vi "IV_Reader.vi"(7 "Path to PNG Folder":path, 8 "Use only a subset of the folder":bool=TRUE, 9 "Subset Length":i32, 10 "Subset Index":i32, 11 "Folder or File":path=path "B:/SketchSET/SA03008H.20180718/08-BG_Sweep_-5to5_0.1_@0.1Hz") -> ()   [LabVIEW 2016]
uses:
  <userlib>/LevyLab/LV to ITX/LVtoITX.lvclass
  <vilib>/Analysis/NI_AALBase.lvlib
  <vilib>/Analysis/1siggen.llb/Ramp Pattern by Delta.vi
  <vilib>/MakerHub/Toolbox/LMH-Toolbox.lvlib
panel:
  in  "dI/dV OFFSET":dbl=100.0 format="%#_13g"
  in  "IV OFFSET":dbl=2e-10 format="%#_13g"
  in  "e^2/h ?":bool
  in  "X step":dbl
  in  "X start":dbl
  out "Differential Conductance":dbl[][](graph)=[[172.002], [172.014], [172.02], [172.032], [172.05], [172.038], [171.99], [171.984], [172.008], [172.02], [172.038], [172.032], [172.008], [171.99], [171.984], [171.99], [172.008], [172.02], [172.032], [171.996], [172.002], [172.014], [172.032], [172.056], [172.056], [172.038], [172.008], [171.996], [172.014], [172.026], [172.032], [172.044], [172.008], [171.996], [171.99], [172.014], [172.032], [172.038], [172.032], [171.99], [171.984], [171.996], [172.014], [172.032], [172.026], [172.002], [171.99], [171.996], [172.02], [172.038], [172.05], [172.032], [172.002], [172.008], [172.014], [172.032], [172.044], [172.056], [172.044], [172.002], [171.996], [172.002], [172.026], [172.038], [172.044], [172.05], [172.02], [172.002], [171.99], [172.002], [172.008], [172.026], [172.02], [171.978], [171.978], [171.984], [171.99], [171.99], [172.002], [171.978], [171.96], [171.972], [171.984], [171.99], [171.996], [171.996], [171.978], [171.954], [171.948], [171.972], [171.99], [172.008], [172.032], [172.014], [171.996], [172.008], [172.014], [172.014], [172.008], [171.99], [171.972], [171.972], [171.99], [172.008], [172.032], [172.02], [171.996], [171.984], [171.996], [172.014], [172.02], [172.002], [171.972], [171.978], [171.99], [172.008], [172.026], [172.026], [171.99], [171.978], [171.99], [171.996], [172.002], [172.002], [172.002]]
  in  "Portion of data":cluster{dbl, dbl}(slide)={0.75, 0.25} scale=0.0..1.0
  out "hmmmm":cluster{dbl[], dbl[]}(graph)
  out "Iterations of loop":i32
  out "directory":bool
  out "dI/dV":cluster{dbl[], dbl[]}[](graph)
  out "A vs B":cluster{dbl[], dbl[]}[](graph)
  in  "Diff bin size":dbl
  out "Comments":string
  in  "Diff bin size":dbl=2.0
  out "N__":cluster{"N1":dbl, "N2":dbl, "N3":dbl, "N4":dbl}={"N1"=0.0624995231628418, "N2"=0.0624995231628418, "N3"=0.0624995231628418, "N4"=0.0624995231628418} {"N4" format="%#_6p"; "N3" format="%#_6p"; "N2" format="%#_6p"; "N1" format="%#_6p"}
  out "IV":dbl[][](graph)=[[172.002], [172.014], [172.02], [172.032], [172.05], [172.038], [171.99], [171.984], [172.008], [172.02], [172.038], [172.032], [172.008], [171.99], [171.984], [171.99], [172.008], [172.02], [172.032], [171.996], [172.002], [172.014], [172.032], [172.056], [172.056], [172.038], [172.008], [171.996], [172.014], [172.026], [172.032], [172.044], [172.008], [171.996], [171.99], [172.014], [172.032], [172.038], [172.032], [171.99], [171.984], [171.996], [172.014], [172.032], [172.026], [172.002], [171.99], [171.996], [172.02], [172.038], [172.05], [172.032], [172.002], [172.008], [172.014], [172.032], [172.044], [172.056], [172.044], [172.002], [171.996], [172.002], [172.026], [172.038], [172.044], [172.05], [172.02], [172.002], [171.99], [172.002], [172.008], [172.026], [172.02], [171.978], [171.978], [171.984], [171.99], [171.99], [172.002], [171.978], [171.96], [171.972], [171.984], [171.99], [171.996], [171.996], [171.978], [171.954], [171.948], [171.972], [171.99], [172.008], [172.032], [172.014], [171.996], [172.008], [172.014], [172.014], [172.008], [171.99], [171.972], [171.972], [171.99], [172.008], [172.032], [172.02], [171.996], [171.984], [171.996], [172.014], [172.02], [172.002], [171.972], [171.978], [171.99], [172.008], [172.026], [172.026], [171.99], [171.978], [171.99], [171.996], [172.002], [172.002], [172.002]]
  in  "index":T1={"A"=5, "B"=3, "C"=2, "D"=0, "E"=3, "N1"=0, "N2"=0, "N3"=0, "N4"=0}
  # "YES"
  # "NO"
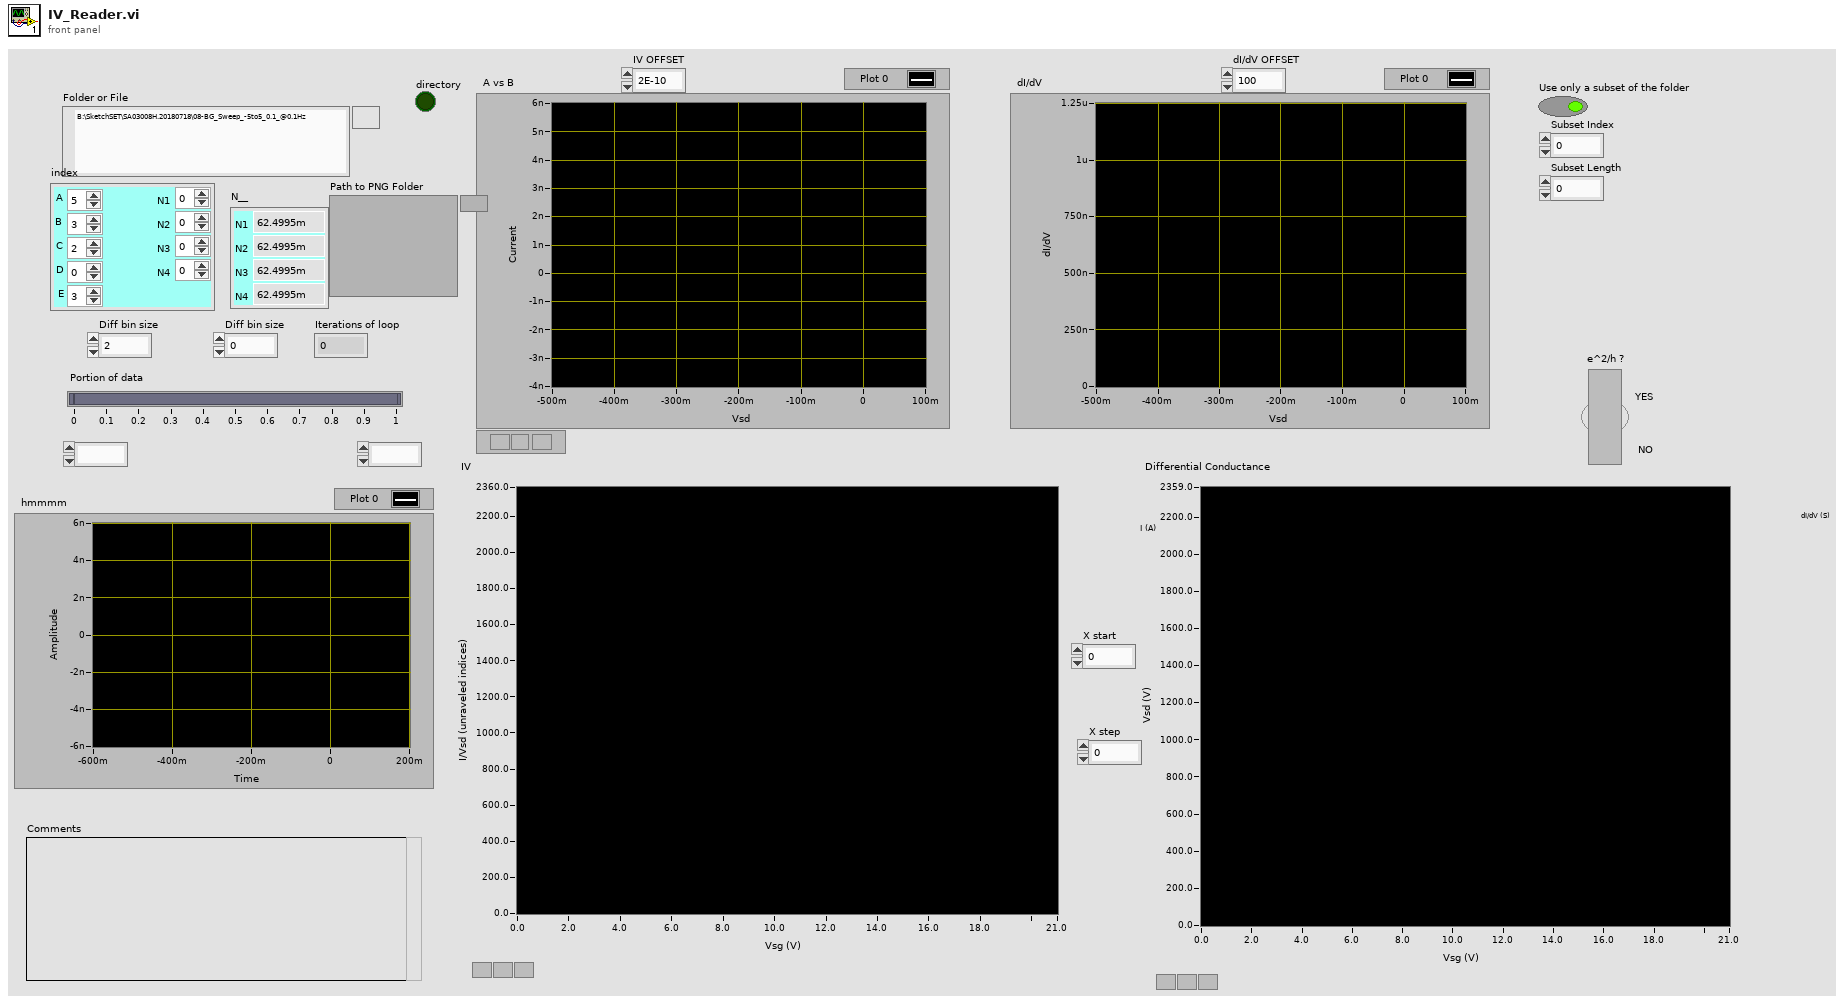
[diagram p1: front panel]
types:
  T1 = cluster{"A":i32, "B":i32, "C":i32, "D":i32, "E":i32, "N1":i32, "N2":i32, "N3":i32, "N4":i32}
  T2 = cluster{"Decimated Array":dbl[], "Decimated Array":dbl[]}[]
  T3 = cluster{"Decimated Array":dbl[], "Decimated Array":dbl[]}
  T4 = typedef "imagedata.ctl" = cluster{"image type":i32, "image depth":i32, "image":u8[], "mask":u8[], "colors":u32[], "Rectangle":cluster{"left":i16, "top":i16, "right":i16, "bottom":i16}}
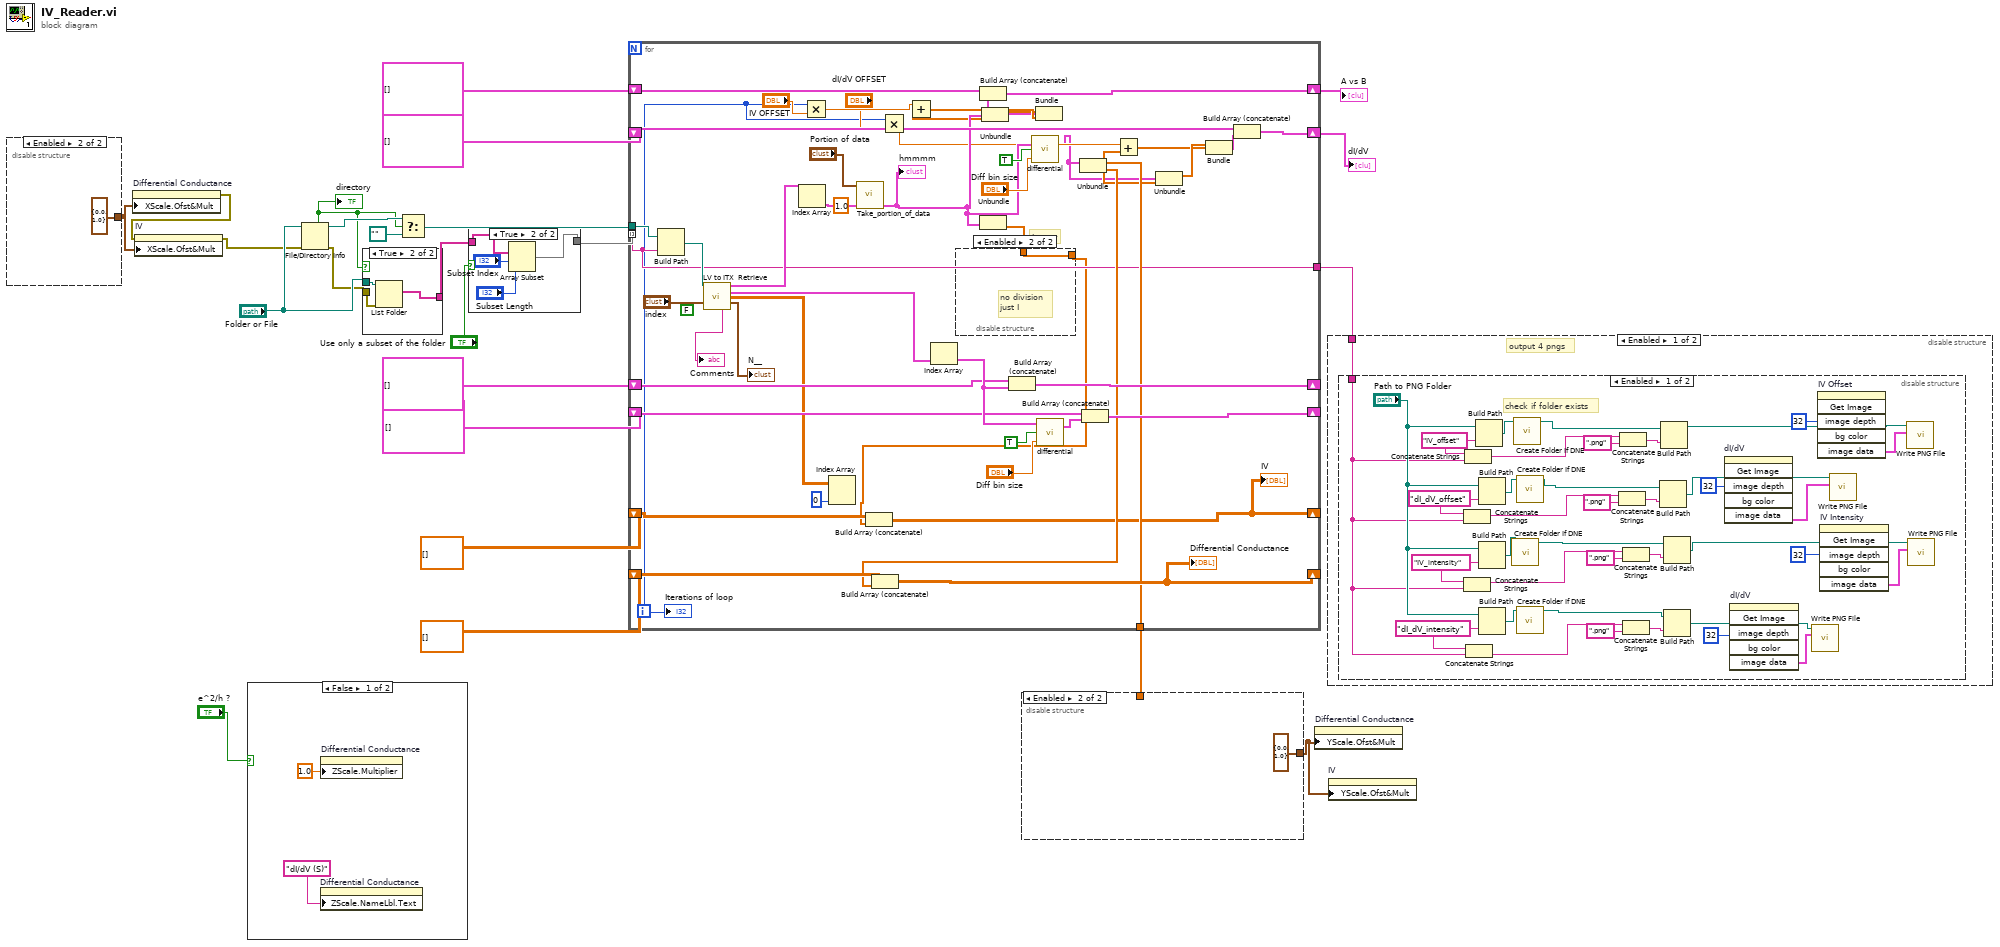
[diagram p0: block diagram]
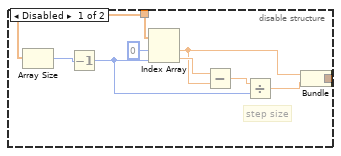
[diagram p5: hidden frame]
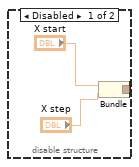
[diagram p6: hidden frame]
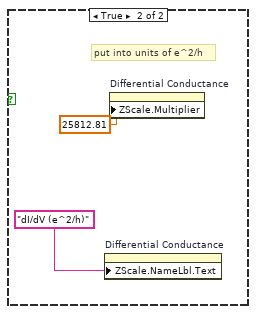
[diagram p7: hidden frame]
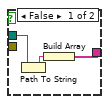
[diagram p8: hidden frame]
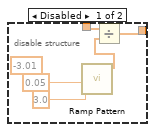
[diagram p9: hidden frame]
diagram:
  n1 = disable-structure shown="Enabled" {
    disable-tunnel: [w25 cluster{"X start":dbl, "X step":dbl} {"X start"=0.0, "X step"=1.0}] -> w11
    frame Disabled {
      n2 = Bundle("X start"="X start", "X step"="X step") -> (w25:cluster{"X start":dbl, "X step":dbl})  [unwired: 1 in]
    }
    frame Enabled {
    }
  }
  n3 = property on="Differential Conductance" class="IntGraph (strict)"("XScale.Ofst&Mult"=w11) -> (error out=w9:errorcluster)  [unwired: 2 in, 1 out]
  n4 = property on="IV" class="IntGraph (strict)"(error in=w9, "XScale.Ofst&Mult"=w11) -> (error out=w8:errorcluster)  [unwired: 1 in, 1 out]
  n5 = case shown="False" "e^2/h ?" {
    frame False {
      n6 = property on="Differential Conductance" class="IntGraph (strict)"("ZScale.Multiplier"=1.0 ("Z Scale.Offset and Multiplier:Multiplier")) -> ()  [unwired: 2 in, 2 out]
      n7 = property on="Differential Conductance" class="IntGraph (strict)"("ZScale.NameLbl.Text"="dI/dV (S)" ("Z Scale.Unit Label.Text")) -> ()  [unwired: 2 in, 2 out]
    }
    frame True {
      # "put into units of e^2/h"
      n8 = property on="Differential Conductance" class="IntGraph (strict)"("ZScale.NameLbl.Text"="dI/dV (e^2/h)" ("Z Scale.Unit Label.Text")) -> ()  [unwired: 2 in, 2 out]
      n9 = property on="Differential Conductance" class="IntGraph (strict)"("ZScale.Multiplier"=25812.81 ("Z Scale.Offset and Multiplier:Multiplier")) -> ()  [unwired: 2 in, 2 out]
    }
  }
  n10 = File/Directory Info(path="Folder or File", error in=w8) -> (path out=w17:path, directory=w16:bool, error out=w18:errorcluster)  [unwired: 4 out]
  "directory" <- w16
  n11 = case shown="True" w16 {
    tunnel: "Folder or File" -> [w35 w38]
    tunnel: w18 -> [_ w37]
    tunnel: [w33 w36] -> w3
    frame False {
      n12 = Path To String(path=w35) -> (string=w34:string)
      n13 = Build Array(w34) -> (w33:string[])
    }
    frame True {
      n14 = List Folder(path=w38, error in=w37) -> (filenames=w36:string[])  [unwired: 2 in, 3 out]
    }
  }
  n15 = Select(t=w17, s=w16, f=path "") -> (s? t:f=w15:path)
  n16 = case shown="True" "Use only a subset of the folder" {
    tunnel: w3 -> [w39 w43]
    tunnel: [w39 w42] -> w2
    frame False {
    }
    frame True {
      n17 = Array Subset(array=w43, index="Subset Index", length="Subset Length") -> (w42:string[])
    }
  }
  n18 = for {
    shift-right: [w63] -> w4
    shift-left: cluster{dbl[], dbl[]}[] [] -> [w87]
    shift-right: [w62] -> w5
    shift-left: T2 [] -> [w86]
    shift-right: [w77] -> _
    shift-left: T2 [] -> [w81]
    shift-right: [w78] -> _
    shift-left: cluster{dbl[], dbl[]}[] [] -> [w80]
    tunnel: w2 -> [w64] mode=indexing
    shift-right: [w61] -> _
    shift-left: dbl[][] [] -> [w74]
    tunnel: w15 -> [w73]
    shift-right: [w66] -> _
    shift-left: dbl[][] [] -> [w68]
    tunnel: [w65] -> w12
    tunnel: [w64] -> w6
    i -> [w46]
    (unwired) 1.0 ("Decimate point")
    (unwired) FALSE ("stop")
    # "I array"
    n19 = Build Path(base path=w73, name or relative path=w64) -> (appended path=w79:path)
    n20 = call <userlib>:"LV to ITX  Retrieve.vi"("File or Folder Path"=w79, "index"="index") -> ("A vs B"=w70:cluster{dbl[], dbl[]}[], "C vs D"=w72:cluster{dbl[], dbl[]}[], "E"=w76:dbl[][], "N"=→"N__":cluster{"N1":dbl, "N2":dbl, "N3":dbl, "N4":dbl}, "Comments"=→"Comments":string)  [unwired: 9 in]
    n21 = Index Array(array=w70) -> (element=w69:cluster{dbl[], dbl[]})  [unwired: 1 in]
    n22 = Multiply(x=w46, y="IV OFFSET") -> (x*y=w54:dbl)
    n23 = Index Array(array=w76, index (col)=0 ("index (row)")) -> ()  [unwired: 1 in, 1 out]
    n24 = call <userlib>:"Take_portion_of_data.vi"("input IV"=w69, "Slide"="Portion of data") -> ("Output IV"=w60:cluster{dbl[], dbl[]})  [unwired: 5 in]
    "hmmmm" <- w60
    n25 = Multiply(x=w46, y="dI/dV OFFSET") -> (x*y=w53:dbl)
    n26 = Index Array(array=w72) -> (element=w84:cluster{dbl[], dbl[]})  [unwired: 1 in]
    n27 = Unbundle(w60) -> (w45:dbl[])  [unwired: 1 out]
    n28 = disable-structure shown="Enabled" {
      disable-tunnel: w45 -> [w95 w99]
      disable-tunnel: [w93 w99] -> w44
      frame Disabled {
        n29 = call-poly <vilib>:"Ramp Pattern.vi"("start"=-3.01, "end"=3.0, "delta"=0.05) -> ("Ramp Pattern"=w94:dbl[])  [unwired: 6 in, 2 out]
        n30 = Divide(x=w95, y=w94) -> (x/y=w93:dbl[])
      }
      frame Enabled {
        # "no division\njust I"
      }
    }
    n31 = Build Array (concatenate)(w74, w44) -> (w61:dbl[][])
    "IV" <- w61
    n32 = Unbundle(w60) -> (w56:dbl[], w57:dbl[])
    n33 = Add(x=w54, y=w57) -> (x+y=w58:dbl[])
    n34 = Build Array (concatenate)(w80, w84) -> (w78:cluster{dbl[], dbl[]}[])
    n35 = call <userlib>:"differential.vi"("Numeric"="Diff bin size", "dy/dx vs x"=TRUE, "A vs B 2"=w60) -> ("A vs B 3"=w48:T3)  [unwired: 1 in]
    n36 = Bundle(w56, w58) -> (w55:cluster{dbl[], dbl[]})  [unwired: 1 in]
    n37 = Build Array (concatenate)(w87, w55) -> (w63:cluster{dbl[], dbl[]}[])
    n38 = call <userlib>:"differential.vi"("Numeric"="Diff bin size", "dy/dx vs x"=TRUE, "A vs B 2"=w84) -> ("A vs B 3"=w85:T3)  [unwired: 1 in]
    n39 = Unbundle(w48) -> ("Decimated Array"=w65:dbl[], "Decimated Array"=w67:dbl[])
    n40 = Build Array (concatenate)(w68, w67) -> (w66:dbl[][])
    "Differential Conductance" <- w66
    n41 = Build Array (concatenate)(w81, w85) -> (w77:T2)
    n42 = Unbundle(w48) -> ("Decimated Array"=w50:dbl[], "Decimated Array"=w51:dbl[])
    n43 = Add(x=w53, y=w51) -> (x+y=w47:dbl[])
    n44 = Bundle("Decimated Array"=w50, w47) -> (w49:cluster{"Decimated Array":dbl[], dbl[]})  [unwired: 1 in]
    n45 = Build Array (concatenate)(w86, w49) -> (w62:T2)
    "Iterations of loop" <- w46
  }
  "dI/dV" <- w5
  "A vs B" <- w4
  n46 = disable-structure shown="Enabled" {
    disable-tunnel: w12 -> [w107 _]
    disable-tunnel: [w100 cluster{dbl, dbl} {0.0, 1.0}] -> w10
    frame Disabled {
      # "step size"
      n47 = Array Size(array=w107) -> (size(s)=w104:i32)
      n48 = Decrement(x=w104) -> (x-1=w103:i32)
      n49 = Index Array(array=w107, index #1=0 ("index"), index #2=w103) -> (element #1=w102:dbl, element #2=w106:dbl)
      n50 = Subtract(x=w106, y=w102) -> (x-y=w105:dbl)
      n51 = Divide(x=w105, y=w103) -> (x/y=w101:dbl)
      n52 = Bundle(w102, w101) -> (w100:cluster{dbl, dbl})  [unwired: 1 in]
    }
    frame Enabled {
    }
  }
  n53 = property on="Differential Conductance" class="IntGraph (strict)"("YScale.Ofst&Mult"=w10) -> ()  [unwired: 2 in, 2 out]
  n54 = disable-structure shown="Enabled" {
    disable-tunnel: w6 -> [w110 _]
    frame Enabled {
      # "output 4 pngs"
      n55 = disable-structure shown="Enabled" {
        disable-tunnel: w110 -> [w141 _]
        frame Enabled {
          w142 = "dI_dV_intensity" ("name or relative path")
          w143 = "IV_intensity" ("name or relative path")
          w144 = "dI_dV_offset" ("name or relative path")
          w145 = "IV_offset" ("name or relative path")
          # "check if folder exists"
          n56 = Concatenate Strings(w144, w141) -> (w131:string)
          n57 = Concatenate Strings(w143, w141) -> (w132:string)
          n58 = Concatenate Strings(w145, w141) -> (w140:string)
          n59 = Concatenate Strings(w142, w141) -> (w133:string)
          n60 = Build Path(base path="Path to PNG Folder", name or relative path=w145) -> (appended path=w118:path)
          n61 = Build Path(base path="Path to PNG Folder", name or relative path=w144) -> (appended path=w111:path)
          n62 = Build Path(base path="Path to PNG Folder", name or relative path=w143) -> (appended path=w114:path)
          n63 = Build Path(base path="Path to PNG Folder", name or relative path=w142) -> (appended path=w116:path)
          n64 = call <vilib>:"Create Folder If DNE.vi"("Folder Path"=w114) -> ("Dup Path"=w113:path)  [unwired: 9 in, 1 out]
          n65 = call <vilib>:"Create Folder If DNE.vi"("Folder Path"=w118) -> ("Dup Path"=w117:path)  [unwired: 9 in, 1 out]
          n66 = call <vilib>:"Create Folder If DNE.vi"("Folder Path"=w111) -> ("Dup Path"=w112:path)  [unwired: 9 in, 1 out]
          n67 = call <vilib>:"Create Folder If DNE.vi"("Folder Path"=w116) -> ("Dup Path"=w115:path)  [unwired: 9 in, 1 out]
          n68 = Concatenate Strings(w131, ".png" ("string")) -> (w138:string)
          n69 = Concatenate Strings(w140, ".png" ("string")) -> (w148:string)
          n70 = Concatenate Strings(w132, ".png" ("string")) -> (w137:string)
          n71 = Concatenate Strings(w133, ".png" ("string")) -> (w134:string)
          n72 = Build Path(base path=w112, name or relative path=w138) -> (appended path=w122:path)
          n73 = Build Path(base path=w117, name or relative path=w148) -> (appended path=w130:path)
          n74 = Build Path(base path=w113, name or relative path=w137) -> (appended path=w126:path)
          n75 = Build Path(base path=w115, name or relative path=w134) -> (appended path=w119:path)
          n76 = invoke on="dI/dV" class="XYGraph (strict)" method="Get Image"("image depth"=32 ("Image Depth")) -> ("image data"=w123:T4)  [unwired: 5 in, 5 out]
          n77 = invoke on="dI/dV" class="IntGraph (strict)" method="Get Image"("image depth"=32 ("Image Depth")) -> ("image data"=w120:T4)  [unwired: 5 in, 5 out]
          n78 = call <vilib>:"Write PNG File.vi"("image data"=w120, "path to PNG file"=w119) -> ()  [unwired: 8 in, 2 out]
          n79 = invoke on="IV Offset" class="XYGraph (strict)" method="Get Image"("image depth"=32 ("Image Depth")) -> ("image data"=w128:T4)  [unwired: 5 in, 5 out]
          n80 = invoke on="IV Intensity" class="IntGraph (strict)" method="Get Image"("image depth"=32 ("Image Depth")) -> ("image data"=w127:T4)  [unwired: 5 in, 5 out]
          n81 = call <vilib>:"Write PNG File.vi"("image data"=w123, "path to PNG file"=w122) -> ()  [unwired: 8 in, 2 out]
          n82 = call <vilib>:"Write PNG File.vi"("image data"=w128, "path to PNG file"=w130) -> ()  [unwired: 8 in, 2 out]
          n83 = call <vilib>:"Write PNG File.vi"("image data"=w127, "path to PNG file"=w126) -> ()  [unwired: 8 in, 2 out]
        }
        frame Disabled {
        }
      }
    }
    frame Disabled {
    }
  }
  n84 = property on="IV" class="IntGraph (strict)"("YScale.Ofst&Mult"=w10) -> ()  [unwired: 2 in, 2 out]
